vi "Test sweep.vi"(8 "error in (no error)":errorcluster, 11 "Magna Power in":refnum<class "Magna Power.lvclass">) -> (0 "error out":errorcluster, 3 "Magna Power out":refnum<class "Magna Power.lvclass">)   [LabVIEW 2012, in "Magna Power.lvclass"]
doc: "(Dynamic) A user-level application that simulates the physical front panel of the Instrument. Provide the user with buttons to manually control features of the instrument, and provide indicators of its current state."
uses:
  Magna Power.lvclass
  Fluke Multimeter/Fluke Multimeter.lvclass
  Magna Power.lvclass/Magna Power.ctl
panel:
  in  "Test Sweep":bool
  in  "Zero field":bool
  out "Actual Voltage (V)":dbl
  out "Actual Current (A)":dbl format="%.3f"
  out "Positive?":bool
  out "Status":string
  out "Field (T)":dbl format="%_4g"
  in  "Specify\nCurrent or Field?":bool=TRUE
  in  "Desired Field":dbl format="%.3f"
  in  "Read":bool
  in  "Send to power supply":bool
  in  "stop":bool
  in  "Voltage Limit":dbl=2255.0 format="%.2f"
  in  "Desired Current":dbl format="%.3f"
  in  "On?":bool
  in  "Read Continuously?":bool=TRUE
  in  "Time between reads (ms)":i32
  # "Note: Current/voltage may take 2-3 sec to update\nafter the supply is turned on."
  # "Read from Power Supply"
  # "Power Supply Control"
  # "Max ~ 1.37 T\n(Always positive,\nwill coerce > 1.37)"
  # "Max = 2255 V"
  # "Max ~ 2.184 A"
  # "Magnetic Field"
  # "(Right to left?)"
  # "A positive field corresponds to a north pole located\non the right when looking straight on at magnet"
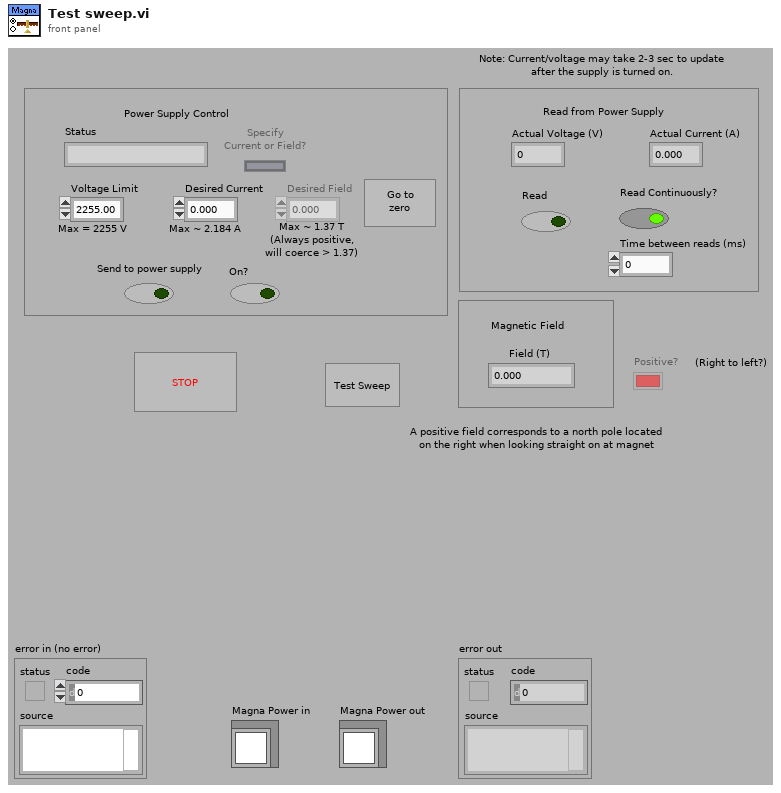
[diagram p1: front panel]
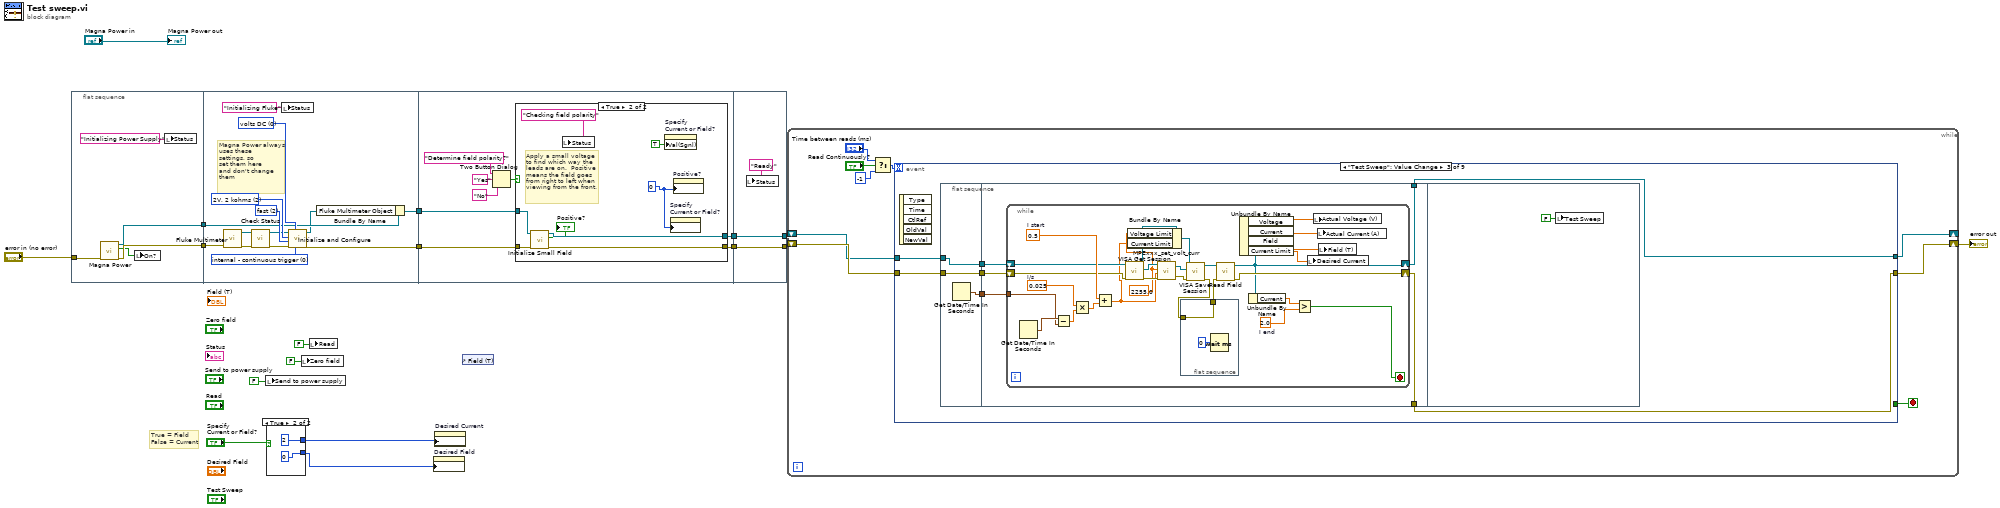
[diagram p0: block diagram]
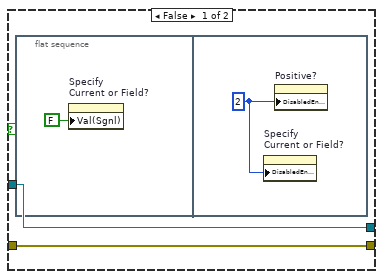
[diagram p2: hidden frame]
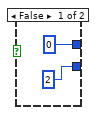
[diagram p3: hidden frame]
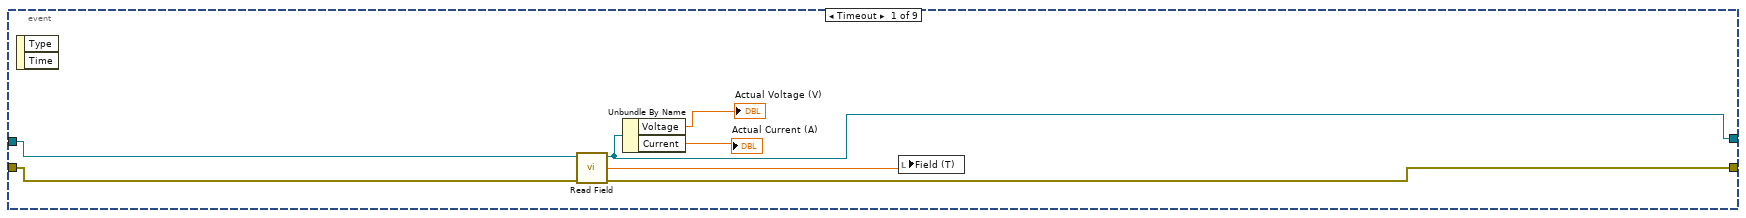
[diagram p4: hidden frame]
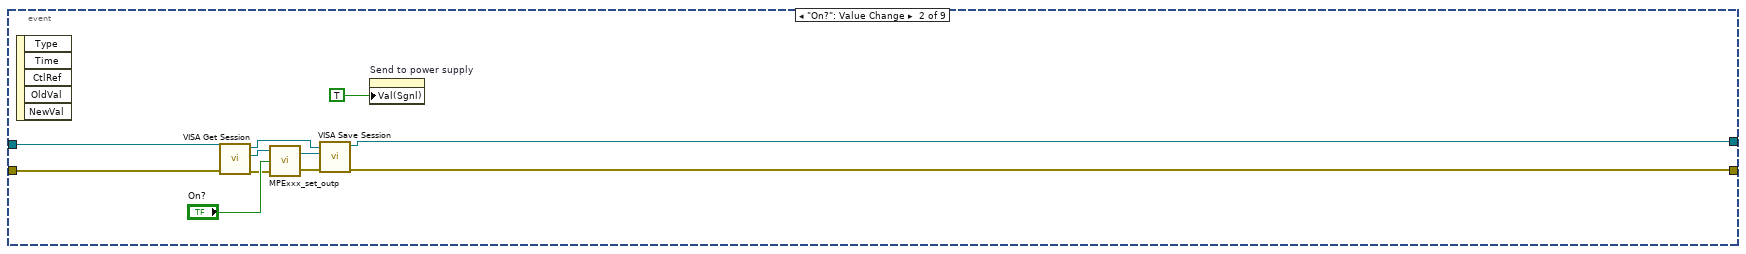
[diagram p5: hidden frame]
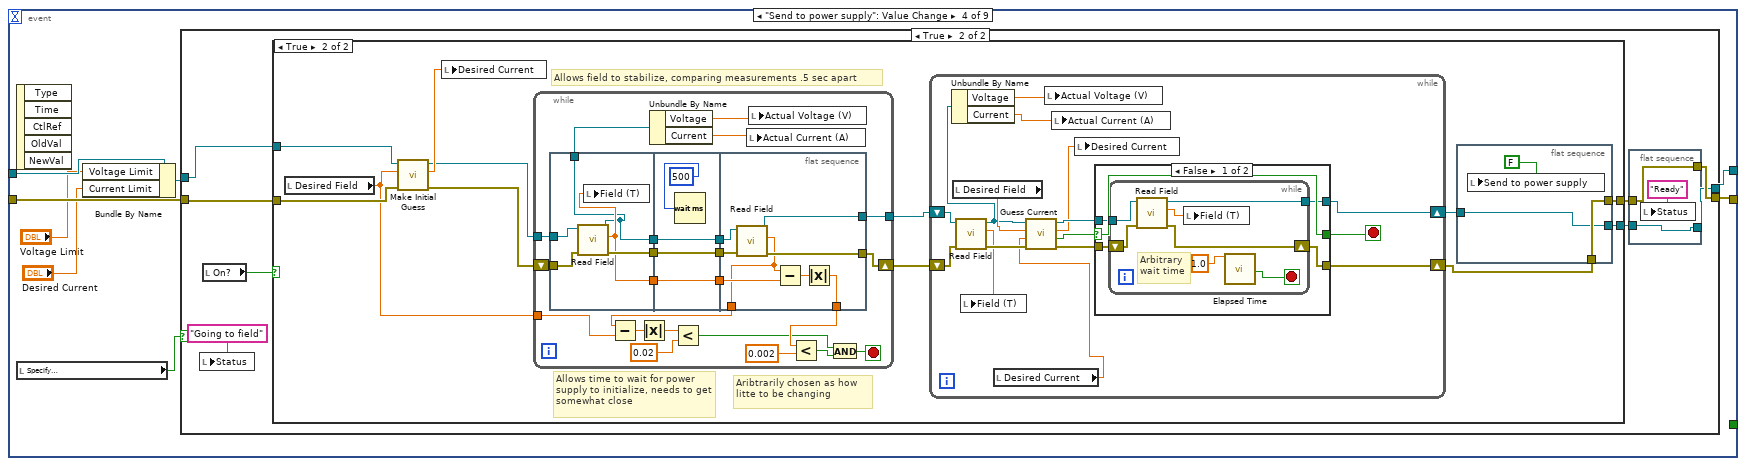
[diagram p6: hidden frame]
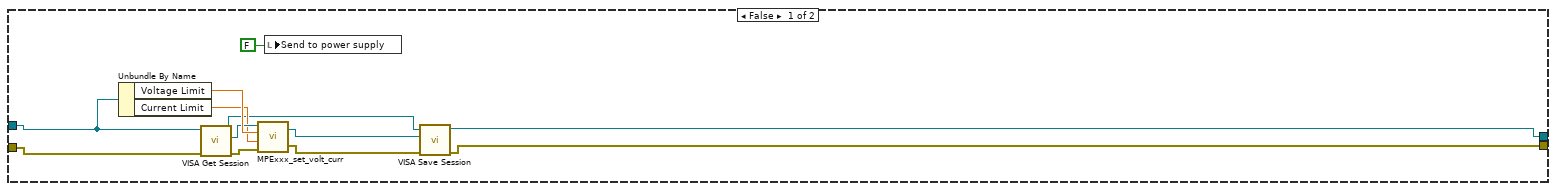
[diagram p7: hidden frame]
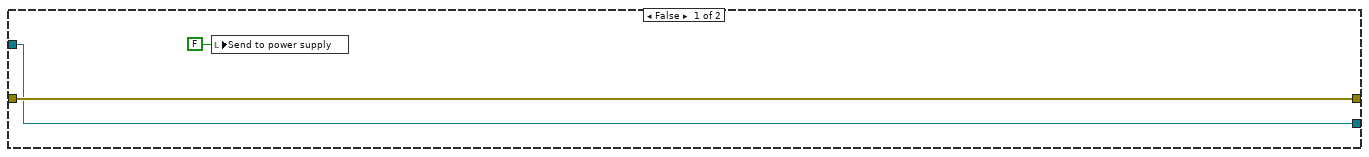
[diagram p8: hidden frame]
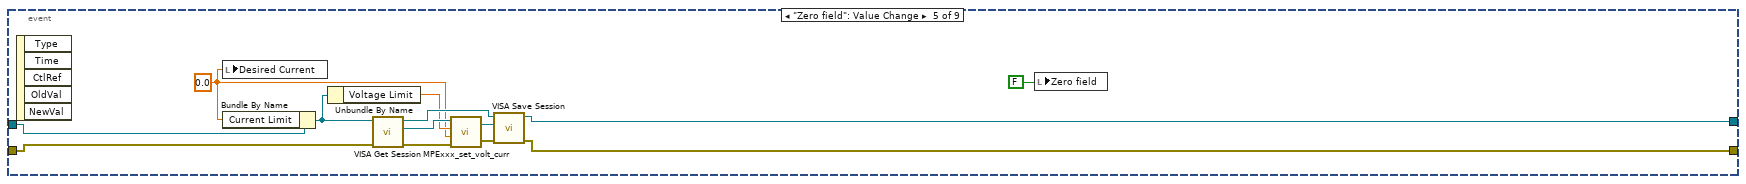
[diagram p10: hidden frame]
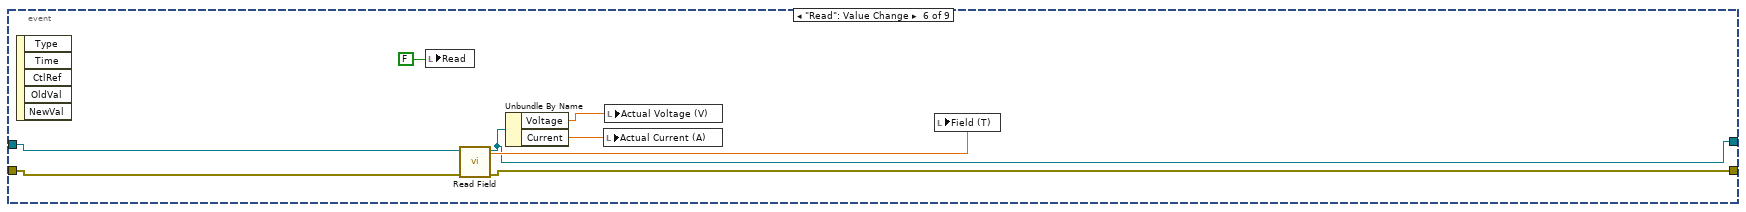
[diagram p11: hidden frame]
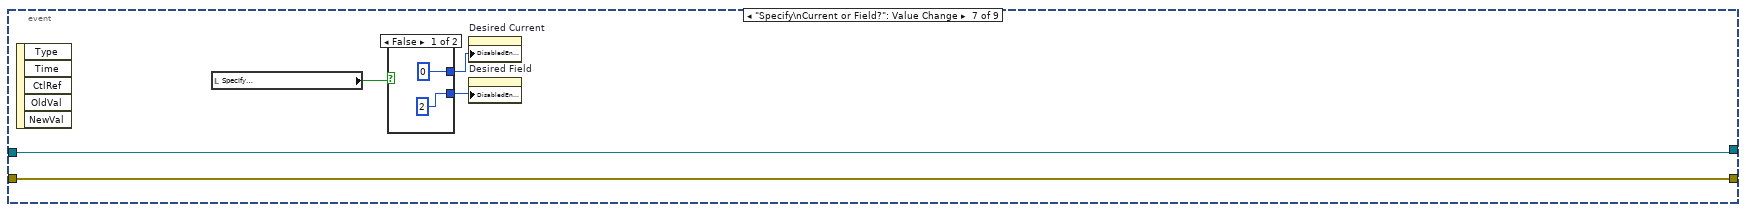
[diagram p12: hidden frame]
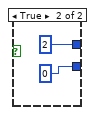
[diagram p13: hidden frame]
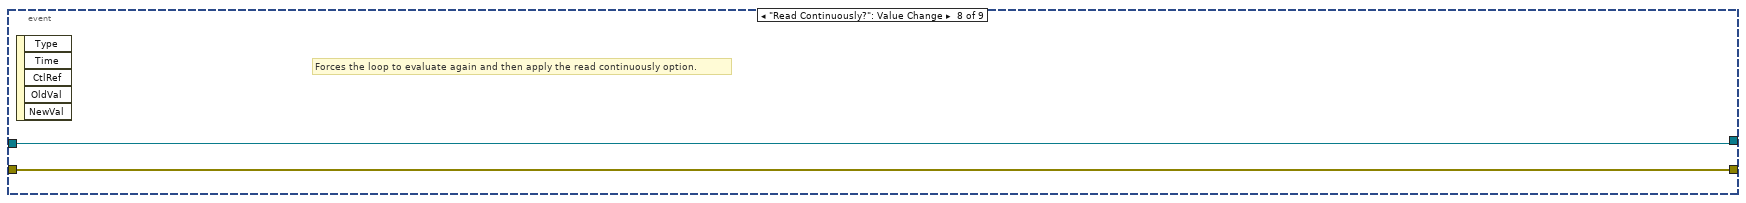
[diagram p14: hidden frame]
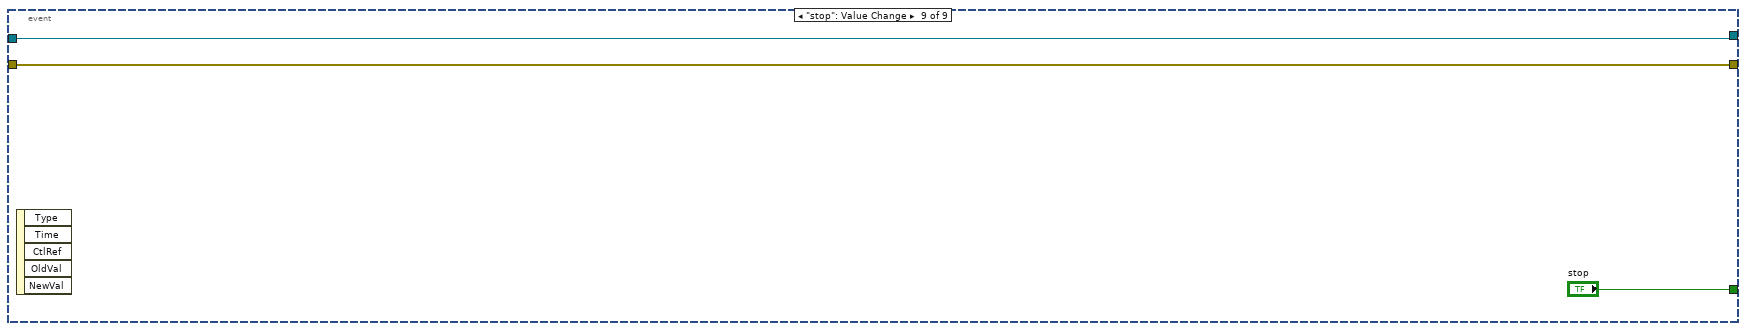
[diagram p15: hidden frame]
diagram:
  # "True = Field\nFalse = Current"
  n1 = flat-sequence {
    tunnel: "error in (no error)" -> [w21]
    tunnel: [w20] -> w16
    tunnel: [w19] -> w6
    tunnel: w16 -> [w30]
    tunnel: [w29] -> w15
    tunnel: w6 -> [w25]
    tunnel: [w23] -> w5
    tunnel: w15 -> [w42]
    tunnel: [w44] -> w14
    tunnel: [w43] -> w13
    tunnel: w5 -> [w37]
    tunnel: [w58] -> w8
    tunnel: [w59] -> w9
    tunnel: w14 -> [w59]
    tunnel: w13 -> [w58]
    frame #0 {
      n2 = call "Magna Power.vi"("error in (no error)"=w21) -> ("error out"=w20:errorcluster, "On?"=w18:bool, "Magna Power out"=w19:refnum<class "Magna Power.lvclass">)  [unwired: 8 in]
      n3 = local write "On?"(w18) -> ()
      n4 = local write "Status"("Initializing Power Supply" ("Status")) -> ()
    }
    frame #1 {
      w36 = u16 0 items=["volts DC", "volts AC", "2-wire k.ohms", "4-wire k.ohms", "mA DC", "mA AC"] ("function (0:volts DC)")
      w35 = u16 2 items=["autorange", "200mV, 200 ohms", "2V, 2 kohms", "20V, 20 kohms", "200V, 200 kohms", "1000Vdc, 700 Vac, 2 Mohms", "20 Mohms", "20 mV, 20 ohms"] ("range (0:auto)")
      w34 = u16 2 items=["slow", "medium", "fast"] ("rate (0:slow)")
      w33 = u16 0 items=["internal - continuous trigger", "external - rear panel trigger with delay", "external - bus trigger with delay", "external - rear panel trigger", "external - bus trigger"] ("trigger mode (0:internal)")
      # "Magna Power always\nuses these\nsettings, so\nset them here\nand don't change\nthem"
      n5 = call "Fluke Multimeter.vi"("error in (no error)"=w30) -> ("error out"=w31:errorcluster, "Fluke Multimeter out"=w27:refnum<class "Fluke Multimeter.lvclass">)  [unwired: 9 in]
      n6 = call-dynamic "Check Status.vi"("error in (no error)"=w31, "Fluke Multimeter in"=w27) -> ("error out"=w32:errorcluster, "Fluke Multimeter out"=w26:refnum<class "Fluke Multimeter.lvclass">)  [unwired: 6 in, 2 out]
      n7 = local write "Status"("Initializing Fluke" ("Status")) -> ()
      n8 = call "Initialize and Configure.vi"("trigger mode (0:internal)"=w33, "function (0:volts DC)"=w36, "error in (no error)"=w32, "rate (0:slow)"=w34, "range (0:auto)"=w35, "Fluke Multimeter.lvclass In"=w26) -> ("error out"=w29:errorcluster, "Fluke Multimeter.lvclass Out"=w24:refnum<class "Fluke Multimeter.lvclass">)  [unwired: 4 in]
      n9 = Bundle By Name(cluster=w25, "Fluke Multimeter Object"=w24) -> (w23:refnum<class "Magna Power.lvclass">)
    }
    frame #2 {
      n10 = Two Button Dialog(message="Determine field polarity?", 1:"No" ("F button name (\"Cancel\")"), 2:"Yes" ("T button name (\"OK\")")) -> (T button?=w41:bool)
      n11 = case shown="True" w41 {
        tunnel: [w45 w56] -> w44
        tunnel: [w46 w55] -> w43
        tunnel: w42 -> [w46 w54]
        tunnel: w37 -> [w45 w49]
        frame False {
          n12 = flat-sequence {
            frame #0 {
              n13 = property on="Specify\nCurrent or Field?" class="Bool (strict)"("Val(Sgnl)"=FALSE ("Value (Signaling)")) -> ()  [unwired: 2 in, 2 out]
            }
            frame #1 {
              w48 = 2
              n14 = property on="Specify\nCurrent or Field?" class="Bool (strict)"("DisabledEnum"=w48) -> ()  [unwired: 2 in, 2 out]
              n15 = property on="Positive?" class="Bool (strict)"("DisabledEnum"=w48) -> ()  [unwired: 2 in, 2 out]
            }
          }
        }
        frame True {
          w51 = 0
          # "Apply a small voltage\nto find which way the\nleads are on.  Positive\nmeans the field goes\nfrom right to left when\nviewing from the front."
          n16 = call "Initialize Small Field.vi"("error in (no error)"=w54, "Magna Power in"=w49) -> ("error out"=w55:errorcluster, "Positive?"=→"Positive?":bool, "Magna Power out"=w56:refnum<class "Magna Power.lvclass">)  [unwired: 7 in]
          n17 = local write "Status"("Checking field polarity" ("Status")) -> ()
          n18 = property on="Specify\nCurrent or Field?" class="Bool (strict)"("Val(Sgnl)"=TRUE ("Value (Signaling)")) -> ()  [unwired: 2 in, 2 out]
          n19 = property on="Specify\nCurrent or Field?" class="Bool (strict)"("DisabledEnum"=w51) -> ()  [unwired: 2 in, 2 out]
          n20 = property on="Positive?" class="Bool (strict)"("DisabledEnum"=w51) -> ()  [unwired: 2 in, 2 out]
        }
      }
    }
    frame #3 {
      n21 = local write "Status"("Ready" ("Status")) -> ()
    }
  }
  n22 = local write "Send to power supply"(FALSE ("Send to power supply")) -> ()
  n23 = case shown="True" "Specify\nCurrent or Field?" {
    tunnel: [2 0] -> w10
    tunnel: [0 2] -> w11
    frame False {
    }
    frame True {
    }
  }
  n24 = local write "Zero field"(FALSE ("Send to power supply")) -> ()
  n25 = local write "Read"(FALSE ("Send to power supply")) -> ()
  n26 = property on="Desired Field" class="DigNum (strict)"("DisabledEnum"=w10) -> ()  [unwired: 2 in, 2 out]
  n27 = property on="Desired Current" class="DigNum (strict)"("DisabledEnum"=w11) -> ()  [unwired: 2 in, 2 out]
  n28 = control-ref of="Field (T)"() -> ()  [unwired: 1 out]
  n29 = while {
    shift-right: [w66] -> w1
    shift-left: w8 -> [w68]
    shift-right: [w64] -> _
    shift-left: w9 -> [w65]
    stop <- w67 stop-if-true
    n30 = Select(t="Time between reads (ms)", s="Read Continuously?", f=-1) -> (s? t:f=w72:i32)
    n31 = event shown="[2] \"Test Sweep\": Value Change" {
      selector: _ -> [_ _ _ _ _ _ _ _ _]
      dyn-events: _ -> [_ _ _ _ _ _ _ _ _]
      timeout: w72 -> [_ _ _ _ _ _ _ _ _]
      tunnel: w65 -> [w78 w84 w97 w140 w268 w274 w278 w287 w289]
      tunnel: w68 -> [w77 w83 w96 w144 w267 w273 w282 w288 w290]
      tunnel: [_ _ _ _ _ _ _ _ "stop"] -> w67
      tunnel: [w76 w81 w91 w143 w258 w276 w282 w288 w290] -> w66
      tunnel: [w75 w80 w92 w141 w257 w272 w278 w287 w289] -> w64
      event Timeout {
        n32 = event-data() -> ()  [unwired: 1 in, 2 out]
        n33 = call "Read Field.vi"("error in (no error)"=w77, "Magna Power in"=w78) -> ("error out"=w76:errorcluster, "Field (T)"=w79:dbl, "Magna Power out"=w75:refnum<class "Magna Power.lvclass">)  [unwired: 7 in]
        n34 = Unbundle By Name(w75) -> ("Voltage"=→"Actual Voltage (V)":dbl, "Current"=→"Actual Current (A)":dbl)
        n35 = local write "Field (T)"(w79) -> ()
      }
      event "On?": Value Change {
        n36 = event-data() -> ()  [unwired: 1 in, 5 out]
        n37 = call-dynamic "VISA Get Session.vi"("error in (no error)"=w83, "Instrument.lvclass in"=w84) -> ("error out"=w88:errorcluster, "VISA Resource Name"=w87:refnum<visa-resource-name>, "Instrument.lvclass out"=w82:refnum<class "Magna Power.lvclass">)  [unwired: 6 in, 1 out]
        n38 = call "MPExxx_set_outp.vi"("error in (no error)"=w88, "Output Control"="On?", "VISA session"=w87) -> ("error out"=w86:errorcluster, "dup VISA session"=w85:refnum<visa-resource-name>)
        n39 = call-dynamic "VISA Save Session.vi"("error in (no error)"=w86, "VISA Resource Name"=w85, "Instrument.lvclass in"=w82) -> ("error out"=w81:errorcluster, "Instrument.lvclass out"=w80:refnum<class "Magna Power.lvclass">)  [unwired: 7 in]
        n40 = property on="Send to power supply" class="Bool (strict)"("Val(Sgnl)"=TRUE) -> ()  [unwired: 2 in, 2 out]
      }
      event "Test Sweep": Value Change {
        n41 = event-data() -> ()  [unwired: 1 in, 5 out]
        n42 = flat-sequence {
          tunnel: w97 -> [w99]
          tunnel: w96 -> [w98]
          tunnel: [w100] -> w95
          tunnel: [w99] -> w94
          tunnel: [w98] -> w93
          tunnel: w95 -> [w105]
          tunnel: w94 -> [w104]
          tunnel: w93 -> [w103]
          tunnel: [w102] -> w92
          tunnel: [w101] -> w91
          frame #0 {
            n43 = Get Date/Time In Seconds() -> (seconds since 1Jan1904=w100:timestamp)
          }
          frame #1 {
            n44 = while {
              tunnel: w105 -> [w132]
              shift-right: [w120] -> w101
              shift-left: w103 -> [w126]
              shift-right: [w116] -> w102
              shift-left: w104 -> [w127]
              stop <- w117 stop-if-true
              w107 = 2255.0 ("Set Current")
              w130 = 0.025  # I/s
              w118 = 2.0  # I end
              w129 = 0.5  # I start
              n45 = Get Date/Time In Seconds() -> (seconds since 1Jan1904=w133:timestamp)
              n46 = Subtract(x=w133, y=w132) -> (x-y=w131:dbl)
              n47 = Multiply(x=w130, y=w131) -> (x*y=w128:dbl)
              n48 = Add(x=w129, y=w128) -> (x+y=w106:dbl)
              n49 = call-dynamic "VISA Get Session.vi"("error in (no error)"=w126, "Instrument.lvclass in"=w127) -> ("error out"=w125:errorcluster, "VISA Resource Name"=w124:refnum<visa-resource-name>, "Instrument.lvclass out"=w111:refnum<class "Magna Power.lvclass">)  [unwired: 6 in, 1 out]
              n50 = Bundle By Name(cluster=w111, "Voltage Limit"=w107, "Current Limit"=w106) -> (w110:refnum<class "Magna Power.lvclass">)
              n51 = call "MPExxx_set_volt_curr.vi"("error in (no error)"=w125, "Set Current"=w106, "Set Voltage"=w107, "VISA session"=w124) -> ("error out"=w122:errorcluster, "dup VISA session"=w123:refnum<visa-resource-name>)
              n52 = flat-sequence {
                tunnel: w109 -> [w134]
                tunnel: [w134] -> w108
                frame #0 {
                  n53 = Wait (ms)(milliseconds to wait=u32 0) -> ()  [unwired: 1 out]
                }
              }
              n54 = call-dynamic "VISA Save Session.vi"("error in (no error)"=w122, "VISA Resource Name"=w123, "Instrument.lvclass in"=w110) -> ("error out"=w109:errorcluster, "Instrument.lvclass out"=w121:refnum<class "Magna Power.lvclass">)  [unwired: 7 in]
              n55 = call "Read Field.vi"("error in (no error)"=w108, "Magna Power in"=w121) -> ("error out"=w120:errorcluster, "Magna Power out"=w116:refnum<class "Magna Power.lvclass">)  [unwired: 7 in, 1 out]
              n56 = Unbundle By Name(w116) -> ("Voltage"=w115:dbl, "Current"=w114:dbl, "Field"=w113:dbl, "Current Limit"=w112:dbl)
              n57 = Unbundle By Name(w116) -> ("Current"=w119:dbl)
              n58 = Greater?(x=w119, y=w118) -> (0:w117:bool)
              n59 = local write "Desired Current"(w112) -> ()
              n60 = local write "Actual Voltage (V)"(w115) -> ()
              n61 = local write "Actual Current (A)"(w114) -> ()
              n62 = local write "Field (T)"(w113) -> ()
            }
          }
          frame #2 {
            n63 = local write "Test Sweep"(FALSE ("Test Sweep")) -> ()
          }
        }
      }
      event "Send to power supply": Value Change {
        n64 = event-data() -> ()  [unwired: 1 in, 5 out]
        n65 = local read "Specify\nCurrent or Field?"() -> (w142:bool)
        n66 = Bundle By Name(cluster=w140, "Voltage Limit"="Voltage Limit", "Current Limit"="Desired Current") -> (w139:refnum<class "Magna Power.lvclass">)
        n67 = case shown="True" w142 {
          tunnel: w139 -> [w145 w163]
          tunnel: w144 -> [w155 w164]
          tunnel: [w150 w160] -> w143
          tunnel: [w152 w158] -> w141
          frame False {
            n68 = Unbundle By Name(w145) -> ("Voltage Limit"=w151:dbl, "Current Limit"=w147:dbl)
            n69 = call-dynamic "VISA Get Session.vi"("error in (no error)"=w155, "Instrument.lvclass in"=w145) -> ("error out"=w154:errorcluster, "VISA Resource Name"=w149:refnum<visa-resource-name>, "Instrument.lvclass out"=w146:refnum<class "Magna Power.lvclass">)  [unwired: 6 in, 1 out]
            n70 = call "MPExxx_set_volt_curr.vi"("error in (no error)"=w154, "Set Current"=w147, "Set Voltage"=w151, "VISA session"=w149) -> ("error out"=w153:errorcluster, "dup VISA session"=w148:refnum<visa-resource-name>)
            n71 = local write "Send to power supply"(FALSE) -> ()
            n72 = call-dynamic "VISA Save Session.vi"("error in (no error)"=w153, "VISA Resource Name"=w148, "Instrument.lvclass in"=w146) -> ("error out"=w150:errorcluster, "Instrument.lvclass out"=w152:refnum<class "Magna Power.lvclass">)  [unwired: 7 in]
          }
          frame True {
            n73 = local write "Status"("Going to field" ("Status")) -> ()
            n74 = local read "On?"() -> (w162:bool)
            n75 = case shown="True" w162 {
              tunnel: w164 -> [w170 w182]
              tunnel: [w170 w178] -> w159
              tunnel: w163 -> [w168 w181]
              tunnel: [w168 w172] -> w157
              frame False {
                n76 = local write "Send to power supply"(FALSE ("Send to power supply")) -> ()
              }
              frame True {
                # "Allows field to stabilize, comparing measurements .5 sec apart"
                # "Allows time to wait for power supply to initialize, needs to get somewhat close"
                # "Aribtrarily chosen as how litte to be changing"
                n77 = local read "Desired Field"() -> (w175:dbl)
                n78 = call "Make Initial Guess.vi"("error in (no error)"=w182, "Desired Field"=w175, "Magna Power in"=w181) -> ("error out"=w173:errorcluster, "First guess"=w180:dbl, "Magna Power out"=w174:refnum<class "Magna Power.lvclass">)  [unwired: 6 in]
                n79 = local write "Desired Current"(w180) -> ()
                n80 = while {
                  shift-right: [w233] -> w179
                  shift-left: w173 -> [w239]
                  tunnel: w174 -> [w231]
                  tunnel: [w228] -> w176
                  tunnel: w175 -> [w224]
                  stop <- w227 stop-if-true
                  n81 = flat-sequence {
                    tunnel: w239 -> [w244]
                    tunnel: [w243] -> w237
                    tunnel: [w242] -> w235
                    tunnel: w231 -> [w241]
                    tunnel: [w240] -> w229
                    tunnel: [w240] -> w219
                    tunnel: [w247] -> w238
                    tunnel: w237 -> [w247]
                    tunnel: [w246] -> w236
                    tunnel: w235 -> [w246]
                    tunnel: [w245] -> w230
                    tunnel: w229 -> [w245]
                    tunnel: w238 -> [w256]
                    tunnel: w236 -> [w254]
                    tunnel: [w253] -> w232
                    tunnel: [w252] -> w233
                    tunnel: w230 -> [w249]
                    tunnel: [w251] -> w228
                    tunnel: [w250] -> w225
                    frame #0 {
                      n82 = call "Read Field.vi"("error in (no error)"=w244, "Magna Power in"=w241) -> ("error out"=w243:errorcluster, "Field (T)"=w242:dbl, "Magna Power out"=w240:refnum<class "Magna Power.lvclass">)  [unwired: 7 in]
                      n83 = local write "Field (T)"(w242) -> ()
                    }
                    frame #1 {
                      n84 = Wait (ms)(milliseconds to wait=u32 500) -> ()  [unwired: 1 out]
                    }
                    frame #2 {
                      n85 = call "Read Field.vi"("error in (no error)"=w256, "Magna Power in"=w249) -> ("error out"=w252:errorcluster, "Field (T)"=w250:dbl, "Magna Power out"=w251:refnum<class "Magna Power.lvclass">)  [unwired: 7 in]
                      n86 = Subtract(x=w250, y=w254) -> (x-y=w255:dbl)
                      n87 = Absolute Value(x=w255) -> (abs(x)=w253:dbl)
                    }
                  }
                  n88 = Subtract(x=w225, y=w224) -> (x-y=w223:dbl)
                  n89 = Absolute Value(x=w223) -> (abs(x)=w222:dbl)
                  n90 = Unbundle By Name(w219) -> ("Voltage"=w218:dbl, "Current"=w217:dbl)
                  n91 = Less?(x=w222, y=0.02) -> (x < y?=w220:bool)
                  n92 = local write "Actual Current (A)"(w217) -> ()
                  n93 = local write "Actual Voltage (V)"(w218) -> ()
                  n94 = Less?(x=w232, y=0.002) -> (x < y?=w226:bool)
                  n95 = And(x=w220, y=w226) -> (x .and. y?=w227:bool)
                }
                n96 = while {
                  shift-right: [w197] -> w177
                  shift-left: w179 -> [w201]
                  shift-right: [w188] -> w171
                  shift-left: w176 -> [w196]
                  stop <- w190 stop-if-true
                  n97 = local read "Desired Field"() -> (w193:dbl)
                  n98 = call "Read Field.vi"("error in (no error)"=w201, "Magna Power in"=w196) -> ("error out"=w200:errorcluster, "Field (T)"=w192:dbl, "Magna Power out"=w189:refnum<class "Magna Power.lvclass">)  [unwired: 7 in]
                  n99 = Unbundle By Name(w189) -> ("Voltage"=w187:dbl, "Current"=w186:dbl)
                  n100 = local write "Field (T)"(w192) -> ()
                  n101 = local read "Desired Current"() -> (w191:dbl)
                  n102 = call "Guess Current.vi"("error in (no error)"=w200, "Current guess"=w191, "Desired Field"=w193, "Magna Power in"=w189) -> ("error out"=w198:errorcluster, "Stop?"=w199:bool, "New guess"=w194:dbl, "Magna Power out"=w195:refnum<class "Magna Power.lvclass">)  [unwired: 4 in]
                  n103 = local write "Actual Voltage (V)"(w187) -> ()
                  n104 = local write "Actual Current (A)"(w186) -> ()
                  n105 = local write "Desired Current"(w194) -> ()
                  n106 = case shown="False" w199 {
                    selector: w199 -> [w205 w216]
                    tunnel: [w205 w216] -> w190
                    tunnel: w198 -> [w206 w215]
                    tunnel: [w204 w215] -> w197
                    tunnel: w195 -> [w203 w214]
                    tunnel: [w202 w214] -> w188
                    frame False {
                      n107 = while {
                        shift-right: [w211] -> w204
                        shift-left: w206 -> [w213]
                        tunnel: w203 -> [w209]
                        tunnel: [w207] -> w202
                        stop <- w208 stop-if-true
                        # "Arbitrary\nwait time"
                        n108 = call "Read Field.vi"("error in (no error)"=w213, "Magna Power in"=w209) -> ("error out"=w211:errorcluster, "Field (T)"=w212:dbl, "Magna Power out"=w207:refnum<class "Magna Power.lvclass">)  [unwired: 7 in]
                        n109 = local write "Field (T)"(w212) -> ()
                        n110 = call "Elapsed Time"("Time Target (s)"=1.0) -> ("Time has Elapsed"=w208:bool)  [unwired: 11 in, 7 out]
                      }
                    }
                    frame True {
                    }
                  }
                }
                n111 = flat-sequence {
                  tunnel: [w184] -> w178
                  tunnel: w177 -> [w184]
                  tunnel: [w183] -> w172
                  tunnel: w171 -> [w183]
                  frame #0 {
                    n112 = local write "Send to power supply"(FALSE) -> ()
                  }
                }
              }
            }
            n113 = flat-sequence {
              tunnel: [w166] -> w160
              tunnel: w159 -> [w166]
              tunnel: [w165] -> w158
              tunnel: w157 -> [w165]
              frame #0 {
                n114 = local write "Status"("Ready" ("Status")) -> ()
              }
            }
          }
        }
      }
      event "Zero field": Value Change {
        w259 = 0.0 ("Desired Current")
        n115 = event-data() -> ()  [unwired: 1 in, 5 out]
        n116 = local write "Desired Current"(w259) -> ()
        n117 = Bundle By Name(cluster=w268, "Current Limit"=w259) -> (w261:refnum<class "Magna Power.lvclass">)
        n118 = Unbundle By Name(w261) -> ("Voltage Limit"=w260:dbl)
        n119 = call-dynamic "VISA Get Session.vi"("error in (no error)"=w267, "Instrument.lvclass in"=w261) -> ("error out"=w266:errorcluster, "VISA Resource Name"=w262:refnum<visa-resource-name>, "Instrument.lvclass out"=w263:refnum<class "Magna Power.lvclass">)  [unwired: 6 in, 1 out]
        n120 = call "MPExxx_set_volt_curr.vi"("error in (no error)"=w266, "Set Current"=w259, "Set Voltage"=w260, "VISA session"=w262) -> ("error out"=w265:errorcluster, "dup VISA session"=w264:refnum<visa-resource-name>)
        n121 = call-dynamic "VISA Save Session.vi"("error in (no error)"=w265, "VISA Resource Name"=w264, "Instrument.lvclass in"=w263) -> ("error out"=w258:errorcluster, "Instrument.lvclass out"=w257:refnum<class "Magna Power.lvclass">)  [unwired: 7 in]
        n122 = local write "Zero field"(FALSE ("Send to power supply")) -> ()
      }
      event "Read": Value Change {
        n123 = event-data() -> ()  [unwired: 1 in, 5 out]
        n124 = local write "Read"(FALSE) -> ()
        n125 = call "Read Field.vi"("error in (no error)"=w273, "Magna Power in"=w274) -> ("error out"=w276:errorcluster, "Field (T)"=w275:dbl, "Magna Power out"=w272:refnum<class "Magna Power.lvclass">)  [unwired: 7 in]
        n126 = Unbundle By Name(w272) -> ("Voltage"=w271:dbl, "Current"=w270:dbl)
        n127 = local write "Actual Current (A)"(w270) -> ()
        n128 = local write "Actual Voltage (V)"(w271) -> ()
        n129 = local write "Field (T)"(w275) -> ()
      }
      event "Specify\nCurrent or Field?": Value Change {
        n130 = event-data() -> ()  [unwired: 1 in, 5 out]
        n131 = local read "Specify\nCurrent or Field?"() -> (w281:bool)
        n132 = case shown="False" w281 {
          tunnel: [2 0] -> w280
          tunnel: [0 2] -> w279
          frame False {
          }
          frame True {
          }
        }
        n133 = property on="Desired Current" class="DigNum (strict)"("DisabledEnum"=w279) -> ()  [unwired: 2 in, 2 out]
        n134 = property on="Desired Field" class="DigNum (strict)"("DisabledEnum"=w280) -> ()  [unwired: 2 in, 2 out]
      }
      event "Read Continuously?": Value Change {
        # "Forces the loop to evaluate again and then apply the read continuously option."
        n135 = event-data() -> ()  [unwired: 1 in, 5 out]
      }
      event "stop": Value Change {
        n136 = event-data() -> ()  [unwired: 1 in, 5 out]
      }
    }
  }
  "error out" <- w1
  "Magna Power out" <- "Magna Power in"
